vi "Orig_Channel Read Write.vi"() -> ()   [LabVIEW 2021, in "Template Test Helpers.lvlib"]
uses:
  <vilib>/CIF Foundation/CIF Core/CIFCore/Common/Typedef/gRPC Reported Plugin Status.ctl
  <vilib>/CIF Foundation/CIF Core/CIFCore/Common/Typedef/Plugin State.ctl
  <vilib>/CIF Foundation/CIF Core/CIFCore/Common/Typedef/Timing Statistics.ctl
  <vilib>/CIF Foundation/CIF Core/CIFCore/Common/Typedef/Timing Stats Base.ctl
  <vilib>/CIF Foundation/CIF Core/CIFCore/Common/Typedef/FIFO Statistics.ctl
  <vilib>/CIF Foundation/CIF Core/CIFCore/Common/Typedef/Simple Error.ctl
  <vilib>/CIF Foundation/CIF Core/CIFCore/Common/Typedef/Monitor Doubles.ctl
  <vilib>/CIF Foundation/CIF Core/CIFCore/Common/Typedef/Monitor U64.ctl
  <vilib>/CIF Foundation/CIF Core/CIFCore/Common/Typedef/Monitor I64.ctl
  <vilib>/CIF Foundation/CIF Channels Core/CIFChannels/Typedef/Direction.ctl
  <vilib>/CIF Foundation/CIF Core/CIFCore/Grpc/CIFCoreChannel_client/RPC Messages/cif_channelcore_ConnectSubscriber.ctl
  <vilib>/gRPC/LabVIEW gRPC Library/Client API/Close Client.vi
  <vilib>/CIF Foundation/CIF Channels Core/CIPC_Channels/Double/CIF_CIPC_Chn_Double.lvclass
  <vilib>/CIF Foundation/CIF Channels Core/CIPC_Channels/U64/CIF_CIPC_Chn_U64.lvclass
  Template Test Helpers.lvlib
  <vilib>/CIF Foundation/CIF Channels Core/CIFChannels/CIFChannels.lvclass
  <vilib>/CIF Foundation/CIF Core/CIFCore/Grpc/CIFCoreWrapper/CIFCoreWrapper.lvlib
  <vilib>/CIF Foundation/CIF Core/CIFCore/Grpc/CIFCoreChannel_client/CIFCoreChannel_client.lvlib
  <vilib>/CIF Foundation/CIF Core/CIFCore/Class/CIFCorePlugin.lvclass
  Common/Typedef/Channels.ctl
  Common/Template_Common.lvlib
  <vilib>/CIF Foundation/CIF Core/CIFCore/Class/Typedef/Energized States.ctl
  <vilib>/CIF Foundation/CIF Channels Core/ChannelCommon/typedef/New FIFO Instance Response.ctl
  <vilib>/CIF Foundation/CIF Channels Core/ChannelCommon/ChannelCommon.lvlib
  <vilib>/CIF Foundation/CIF Core/Channels/CIFChannelMng/CIFChannelMng.lvclass
  <vilib>/CIF Foundation/CIF Core/CIFCore/Common/CIFCoreCommon.lvlib
panel:
  out "Data 4":u64
  out "error out 4":errorcluster
  out "Node Status":T1 {"Monitor Doubles"."4" format="%#_9g"; "Monitor Doubles"."3" format="%#_9g"; "Monitor Doubles"."2" format="%#_9g"; "Monitor Doubles"."1" format="%#_9g"}
  in  "address":string="192.168.1.160:50051"
  in  "Data 3":dbl
  out "error out 3":errorcluster
  in  "stop":bool
  out "error out":errorcluster
  out "Data 2":dbl
  in  "Data":dbl
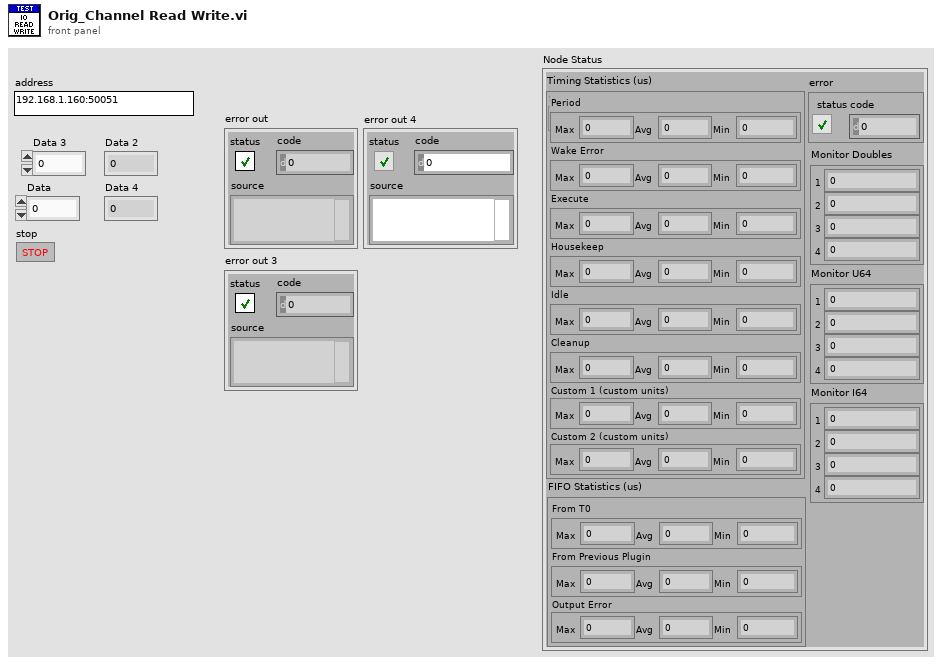
[diagram p1: front panel]
types:
  T1 = typedef "CIFCoreCommon.lvlib/gRPC Reported Plugin Status.ctl" = cluster{"State":T2, "Timing Statistics (us)":T3, "FIFO Statistics (us)":T5, "error":T6, "Monitor Doubles":T7, "Monitor U64":T8, "Monitor I64":T9}
  T2 = typedef "CIFCoreCommon.lvlib/Plugin State.ctl" = enum32{"Null", "Creating", "Listening", "Running", "CleaningUp", "Destroying"}
  T3 = typedef "CIFCoreCommon.lvlib/Timing Statistics.ctl" = cluster{"Period":T4, "Wake Error":T4, "Execute":T4, "Housekeep":T4, "Idle":T4, "Cleanup":T4, "Custom 1 (custom units)":T4, "Custom 2 (custom units)":T4}
  T4 = typedef "CIFCoreCommon.lvlib/Timing Stats Base.ctl" = cluster{"Max":i64, "Avg":dbl, "Min":i64}
  T5 = typedef "CIFCoreCommon.lvlib/FIFO Statistics.ctl" = cluster{"From T0":T4, "From Previous Plugin":T4, "Output Error":T4}
  T6 = typedef "CIFCoreCommon.lvlib/Simple Error.ctl" = cluster{"status":bool, "code":i32}
  T7 = typedef "CIFCoreCommon.lvlib/Monitor Doubles.ctl" = cluster{"1":dbl, "2":dbl, "3":dbl, "4":dbl}
  T8 = typedef "CIFCoreCommon.lvlib/Monitor U64.ctl" = cluster{"1":u64, "2":u64, "3":u64, "4":u64}
  T9 = typedef "CIFCoreCommon.lvlib/Monitor I64.ctl" = cluster{"1":i64, "2":i64, "3":i64, "4":i64}
  T10 = typedef "CIFCoreChannel_client.lvlib/cif_channelcore_ConnectSubscriber.ctl" = cluster{"subscriber_name":string, "publisher_name":string, "custom_connect":u8[]}
  T11 = typedef "CIFChannels.lvclass/Direction.ctl" = enum16{"Publisher", "Subscriber"}
  T12 = typedef "grpc-lvsupport-release.lvlib/grpcId.ctl" = u64
  T13 = typedef "Template_Common.lvlib/Channels.ctl" = enum16{"doubleout", "doublein1", "doublein2", "uint_out", "uint_in", "u8array_out", "u8array_in"}
  T14 = typedef "CIFCorePlugin.lvclass/Energized States.ctl" = enum16{"Listen", "Prepare", "Execute", "Housekeep", "Cleanup", "Destroy"}
  T15 = typedef "ChannelCommon.lvlib/New FIFO Instance Response.ctl" = cluster{"Publisher":string, "Custom Data":u8[]}
  T16 = typedef "Time_CIF_U.lvlib/Clock Conversion Map.ctl" = map{u8, cluster{"Last Reset":i64, "Offset Pair":T17, "Slope":dbl, "1/Slope":dbl}}
  T17 = typedef "Time_CIF_U.lvlib/Timestamp Pair.ctl" = cluster{"System Time":i64, "External Time":i64}
  T18 = typedef "CIFCoreCommon.lvlib/Channel Connection Data.ctl" = cluster{"Publisher Name":string, "Subscriber Name":string, "Connection Data":u8[]}
  T19 = typedef "CIFCoreCommon.lvlib/Channel Force Data.ctl" = cluster{"Channel Name":string, "Force Data":u8[], "Force Active":bool}
  T20 = typedef "CIFCoreCommon.lvlib/FIFO Publisher.ctl" = cluster{"Publisher Name":string, "New FIFO Instance Config":T21}
  T21 = typedef "ChannelCommon.lvlib/New FIFO Instance Configuration.ctl" = cluster{"Backpressure":bool, "Bytes/Message Override":u32, "Messages/FIFO Override":u32, "Custom Data":u8[]}
  T22 = typedef "CIFChannelMng.lvclass/FIFO Publisher Return.ctl" = cluster{"FIFO Instance Config":T15, "error":errorcluster, "Added":bool}
  T23 = typedef "CIFCoreChannel_client.lvlib/cif_channelcore_Channel.ctl" = cluster{"name":string, "direction":T24, "type":string, "custom_config":u8[], "connected":bool, "connected_name":string, "forced":bool, "channel_pattern":T25}
  T24 = typedef "CIFCoreChannel_client.lvlib/cif_channelcore_Direction.ctl" = enum32{"PUBLISHER", "SUBSCRIBER"}
  T25 = typedef "CIFCoreChannel_client.lvlib/cif_channelcore_PATTERN.ctl" = enum32{"UNKNOWN", "TAG", "FIFO", "MULTIFIFO", "BACKPRESSUREFIFO"}
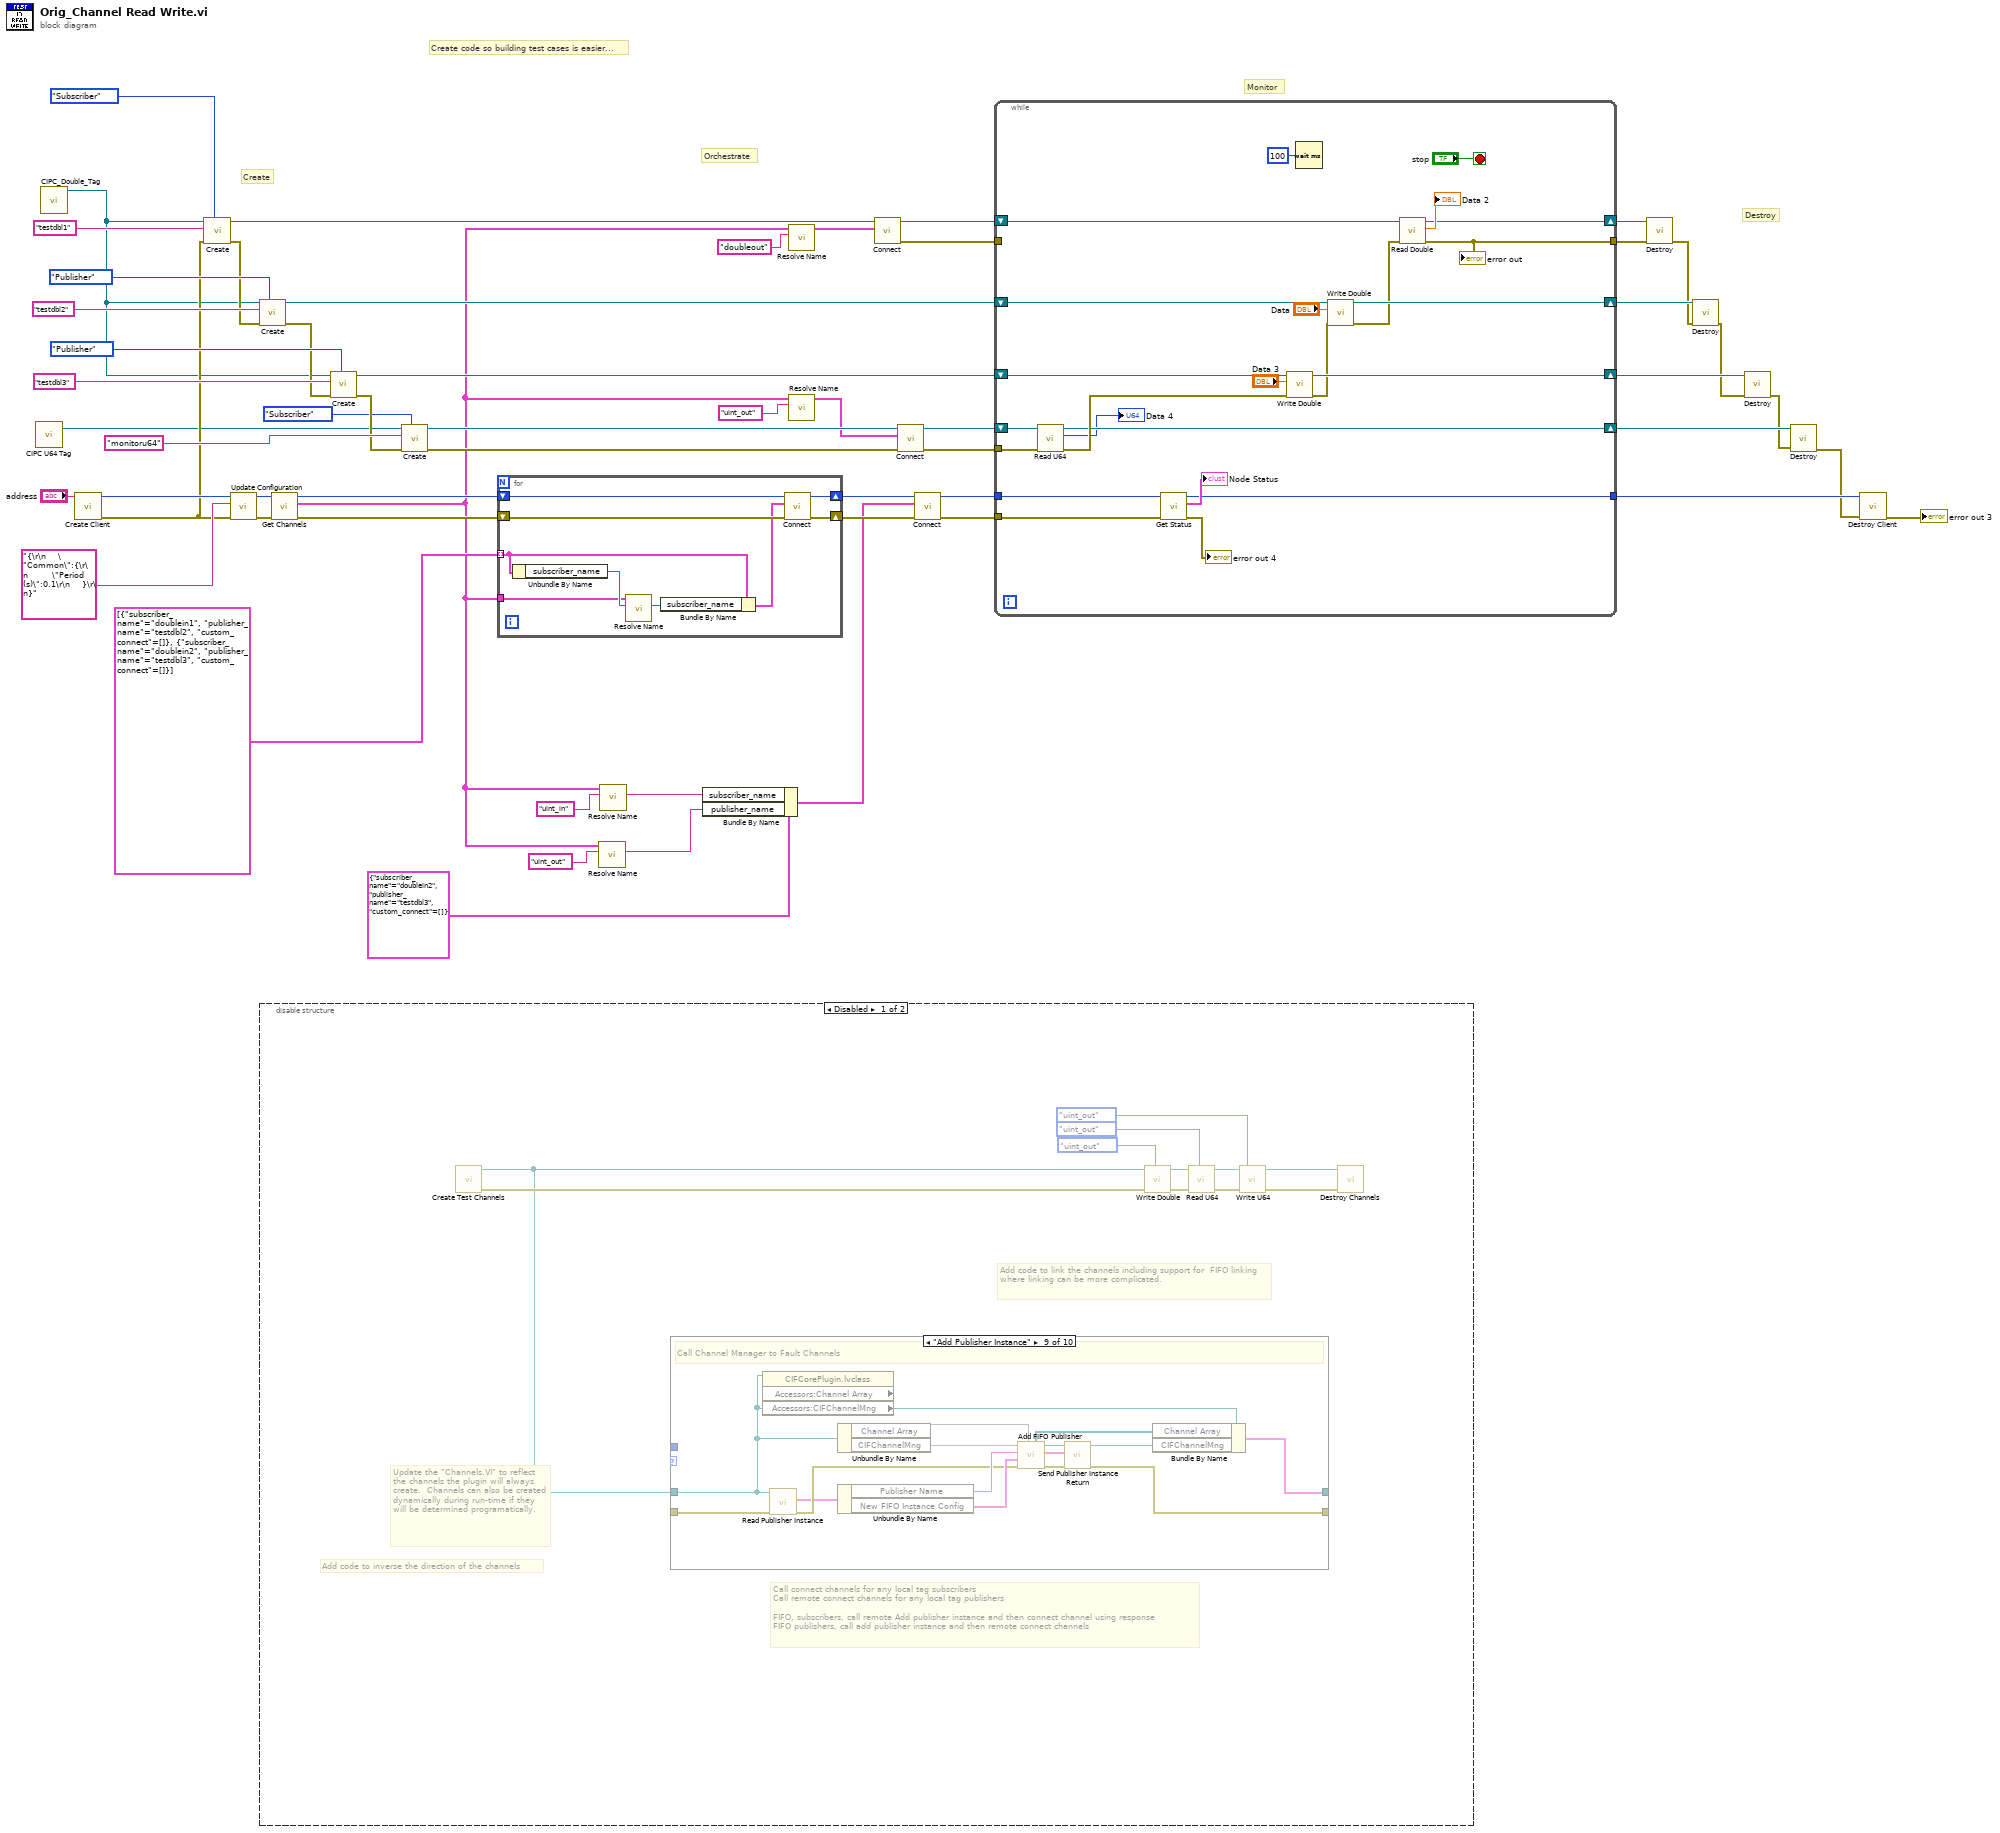
[diagram p0: block diagram]
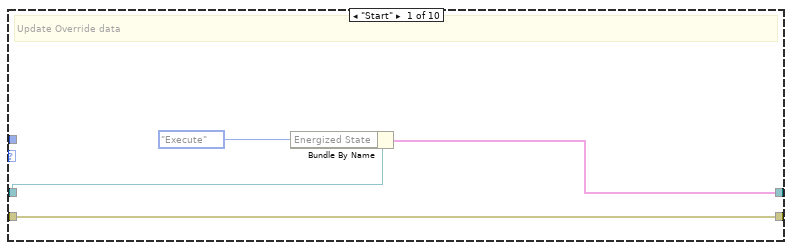
[diagram p2: hidden frame]
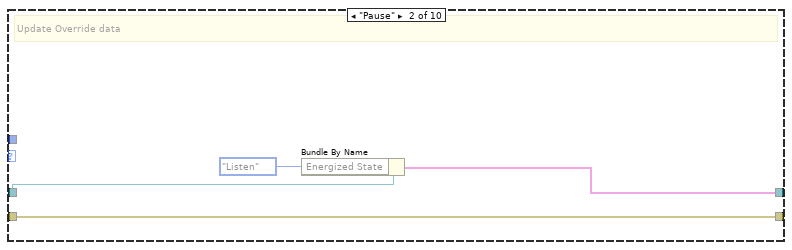
[diagram p3: hidden frame]
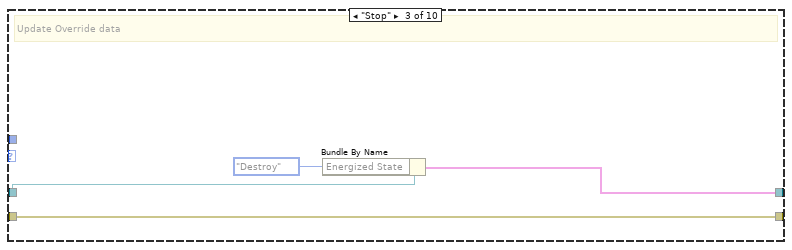
[diagram p4: hidden frame]
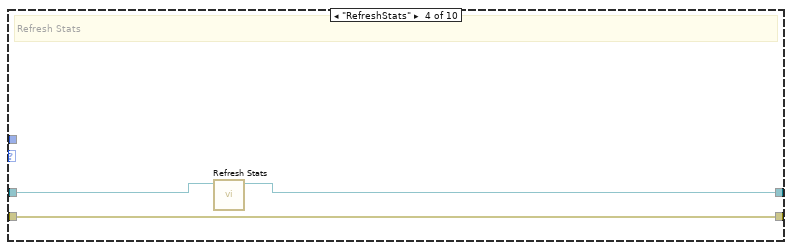
[diagram p5: hidden frame]
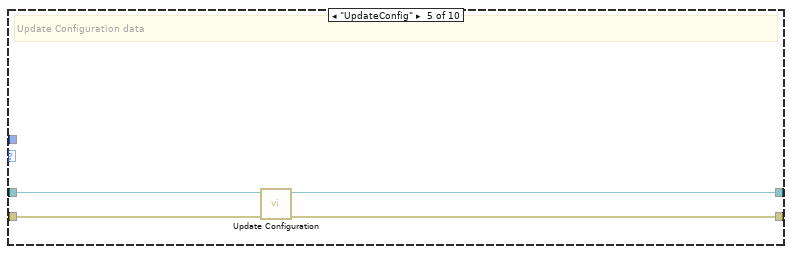
[diagram p6: hidden frame]
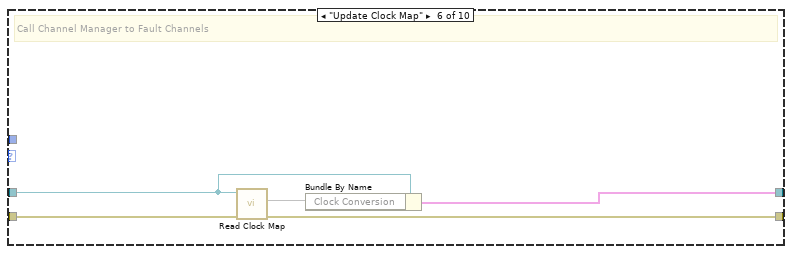
[diagram p7: hidden frame]
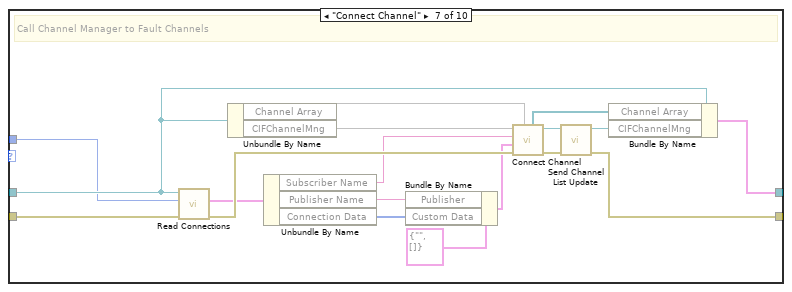
[diagram p8: hidden frame]
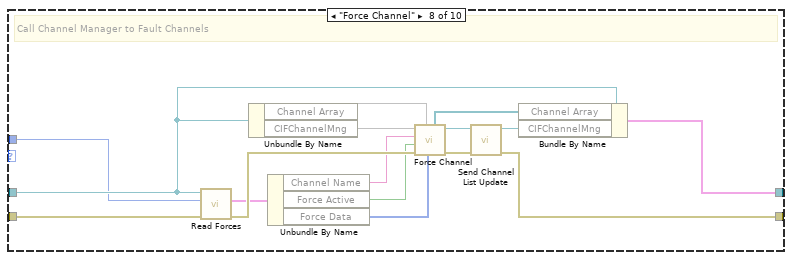
[diagram p9: hidden frame]
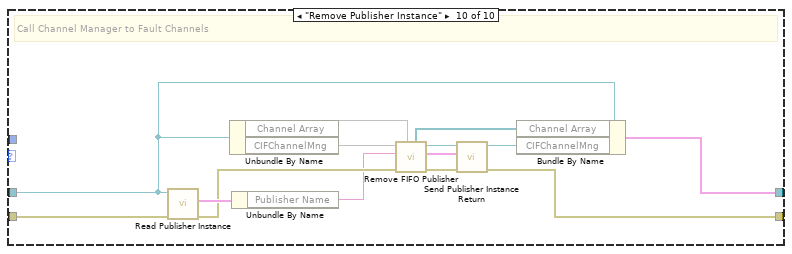
[diagram p10: hidden frame]
diagram:
  # "Create code so building test cases is easier..."
  # "Destroy"
  # "Monitor"
  # "Orchestrate"
  # "Create"
  n1 = call <vilib>:"CIPC U64 Tag.vi"() -> ("CIF_CIPC_Chn_U64.lvclass"=w2:refnum<class "CIF_CIPC_Chn_U64.lvclass">)  [unwired: 11 in]
  n2 = call <vilib>:"CIPC_Double_Tag.vi"() -> ("CIF_CIPC_Chn_Double.lvclass"=w1:refnum<class "CIF_CIPC_Chn_Double.lvclass">)  [unwired: 11 in]
  n3 = call <vilib>:"Create Client.vi"("address"="address") -> ("error out"=w24:errorcluster, "gRPC ID Out"=w25:T12)  [unwired: 9 in]
  n4 = call-dynamic "Create.vi"("Direction"=Direction."Subscriber", "error in (no error)"=w24, "Name"="testdbl1", "CIFTag in"=w1) -> ("error out"=w52:errorcluster, "CIFTag out"=w39:refnum<class "CIF_CIPC_Chn_Double.lvclass">)  [unwired: 6 in]
  n5 = call <vilib>:"Update Configuration.vi"("error in"=w24, "JSON Configuration"="{\r\n    \"Common\":{\r\n        \"Period (s)\":0.1\r\n    }\r\n}" ("JSON Configuration in"), "gRPC ID"=w25) -> ("error out"=w22:errorcluster, "gRPC ID out"=w23:T12)  [unwired: 7 in]
  n6 = call-dynamic "Create.vi"("Direction"=Direction."Publisher", "error in (no error)"=w52, "Name"="testdbl2", "CIFTag in"=w1) -> ("error out"=w43:errorcluster, "CIFTag out"=w55:refnum<class "CIF_CIPC_Chn_Double.lvclass">)  [unwired: 6 in]
  n7 = disable-structure shown="Disabled" {
    frame Disabled {
      # "Call connect channels for any local tag subscribers\nCall remote connect channels for any local tag publishers\n\nFIFO, subscribers, call remote Add publisher instance and then connect channel using response\nFIFO publishers, call add publisher instance and then remote connect channels"
      # "Add code to link the channels including support for  FIFO linking where linking can be more complicated."
      # "Add code to inverse the direction of the channels"
      # "Update the \"Channels.VI\" to reflect the channels the plugin will always create.  Channels can also be created dynamically during run-time if they will be determined programatically."
      n8 = call "Create Test Channels.vi"() -> ("error out"=w68:errorcluster, "CIFCorePlugin out"=w58:refnum<class "CIFCorePlugin.lvclass">)  [unwired: 10 in]
      n9 = case shown="\"Add Publisher Instance\"" {
        selector: _ -> [_ _ _ _ _ _ _ _ _ _]
        tunnel: _ -> [w69 w76 w80 w81 w86 w92 w109 w124 w138 w155]
        tunnel: w58 -> [w70 w75 w79 w83 w87 w88 w101 w113 w127 w142]
        tunnel: [w72 w74 w78 w82 w85 w91 w98 w112 w128 w143] -> _
        tunnel: [w69 w76 w80 w81 w84 w90 w104 w125 w129 w152] -> _
        tunnel: _ -> [_ _ _ _ _ _ w97 w111 _ _]
        frame "Start" {
          # "Update Override data"
          n10 = Bundle By Name(cluster=w70, "Energized State"=Energized_States."Execute" ("Energized States in")) -> (w72:cluster{})
        }
        frame "Pause" {
          # "Update Override data"
          n11 = Bundle By Name(cluster=w75, "Energized State"=Energized_States."Listen" ("Energized States in")) -> (w74:cluster{})
        }
        frame "Stop" {
          # "Update Override data"
          n12 = Bundle By Name(cluster=w79, "Energized State"=Energized_States."Destroy" ("Energized States in")) -> (w78:cluster{})
        }
        frame "RefreshStats" {
          # "Refresh Stats"
          n13 = call <vilib>:"Refresh Stats.vi"("CIFCorePlugin in"=w83) -> ("CIFCorePlugin out"=w82:refnum<class "CIFCorePlugin.lvclass">)  [unwired: 10 in]
        }
        frame "UpdateConfig" {
          # "Update Configuration data"
          n14 = call-dynamic <vilib>:"Update Configuration.vi"("error in (no error)"=w86, "CIFTemplateNode in"=w87) -> ("error out"=w84:errorcluster, "CIFTemplateNode out"=w85:refnum<class "CIFCorePlugin.lvclass">)  [unwired: 8 in]
        }
        frame "Update Clock Map" {
          # "Call Channel Manager to Fault Channels"
          n15 = call <vilib>:"Read Clock Map.vi"("error in"=w92, "CIFCorePlugin in"=w88) -> ("error out"=w90:errorcluster, "Clock Conversion"=w89:T16)  [unwired: 7 in, 1 out]
          n16 = Bundle By Name(cluster=w88, "Clock Conversion"=w89) -> (w91:cluster{})
        }
        frame "Connect Channel" {
          # "Call Channel Manager to Fault Channels"
          n17 = call <vilib>:"Read Connections.vi"("error in"=w109, "index"=w97, "CIFCorePlugin in"=w101) -> ("error out"=w105:errorcluster, "Connection"=w99:T18)  [unwired: 6 in, 1 out]
          n18 = Unbundle By Name(w101) -> ("Channel Array"=w103, "CIFChannelMng"=w110)
          n19 = Unbundle By Name(w99) -> ("Subscriber Name"=w100:string, "Publisher Name"=w95:string, "Connection Data"=w94:u8[])
          n20 = Bundle By Name(cluster=T15 {"Publisher"="", "Custom Data"=[]} ("Connection"), "Publisher"=w95, "Custom Data"=w94) -> (w93:T15)
          n21 = call <vilib>:"Connect Channel.vi"("Channel Array in"=w103, "error in (no error)"=w105, "Connection"=w93, "Subscriber Name"=w100, "CIFChannelMng in"=w110) -> ("error out"=w107:errorcluster, "CIFChannelMng out"=w108:refnum<class "CIFChannelMng.lvclass">, "Channel Array out"=w102:refnum<class "CIFChannels.lvclass">[])  [unwired: 3 in, 1 out]
          n22 = call <vilib>:"Send Channel List Update.vi"("error in (no error)"=w107, "CIFChannelMng in"=w108) -> ("error out"=w104:errorcluster, "CIFChannelMng out"=w106:refnum<class "CIFChannelMng.lvclass">)  [unwired: 8 in]
          n23 = Bundle By Name(cluster=w101, "Channel Array"=w102, "CIFChannelMng"=w106) -> (w98:cluster{})
        }
        frame "Force Channel" {
          # "Call Channel Manager to Fault Channels"
          n24 = call <vilib>:"Read Forces.vi"("error in"=w124, "index"=w111, "CIFCorePlugin in"=w113) -> ("error out"=w122:errorcluster, "Force"=w114:T19)  [unwired: 6 in, 1 out]
          n25 = Unbundle By Name(w113) -> ("Channel Array"=w119, "CIFChannelMng"=w123)
          n26 = Unbundle By Name(w114) -> ("Channel Name"=w117:string, "Force Active"=w116:bool, "Force Data"=w115:u8[])
          n27 = call <vilib>:"Force Channel.vi"("Force Data"=w115, "Channel Array in"=w119, "error in (no error)"=w122, "Force Active"=w116, "Channel Name"=w117, "CIFChannelMng in"=w123) -> ("error out"=w121:errorcluster, "CIFChannelMng out"=w120:refnum<class "CIFChannelMng.lvclass">, "Channel Array out"=w118:refnum<class "CIFChannels.lvclass">[])  [unwired: 2 in, 1 out]
          n28 = call <vilib>:"Send Channel List Update.vi"("error in (no error)"=w121, "CIFChannelMng in"=w120) -> ("error out"=w125:errorcluster, "CIFChannelMng out"=w126:refnum<class "CIFChannelMng.lvclass">)  [unwired: 8 in]
          n29 = Bundle By Name(cluster=w113, "Channel Array"=w118, "CIFChannelMng"=w126) -> (w112:cluster{})
        }
        frame "Add Publisher Instance" {
          # "Call Channel Manager to Fault Channels"
          n30 = property class="CIFCorePlugin.lvclass" props=["Accessors:Channel Array", "Accessors:CIFChannelMng"](reference=w127) -> ()  [unwired: 1 in, 4 out]
          n31 = call <vilib>:"Read Publisher Instance.vi"("error in"=w138, "CIFCorePlugin in"=w127) -> ("error out"=w137:errorcluster, "Publisher Instance"=w136:T20)  [unwired: 7 in, 1 out]
          n32 = Unbundle By Name(w127) -> ("Channel Array"=w132, "CIFChannelMng"=w141)
          n33 = Unbundle By Name(w136) -> ("Publisher Name"=w140:string, "New FIFO Instance Config"=w139:T21)
          n34 = call <vilib>:"Add FIFO Publisher.vi"("Channel Array in"=w132, "error in (no error)"=w137, "New FIFO Instance Config"=w139, "Channel Name"=w140, "CIFChannelMng in"=w141) -> ("error out"=w134:errorcluster, "FIFO Publisher"=w133:T22, "CIFChannelMng out"=w135:refnum<class "CIFChannelMng.lvclass">, "Channel Array out"=w131:refnum<class "CIFChannels.lvclass">[])  [unwired: 2 in, 1 out]
          n35 = call <vilib>:"Send Publisher Instance Return.vi"("error in (no error)"=w134, "Publisher Instance"=w133, "CIFChannelMng in"=w135) -> ("error out"=w129:errorcluster, "CIFChannelMng out"=w130:refnum<class "CIFChannelMng.lvclass">)  [unwired: 7 in]
          n36 = Bundle By Name(cluster=w127, "Channel Array"=w131, "CIFChannelMng"=w130) -> (w128:cluster{})
        }
        frame "Remove Publisher Instance" {
          # "Call Channel Manager to Fault Channels"
          n37 = call <vilib>:"Read Publisher Instance.vi"("error in"=w155, "CIFCorePlugin in"=w142) -> ("error out"=w150:errorcluster, "Publisher Instance"=w154:T20)  [unwired: 7 in, 1 out]
          n38 = Unbundle By Name(w142) -> ("Channel Array"=w145, "CIFChannelMng"=w151)
          n39 = Unbundle By Name(w154) -> ("Publisher Name"=w149:string)
          n40 = call <vilib>:"Remove FIFO Publisher.vi"("Channel Array in"=w145, "error in (no error)"=w150, "Channel Name"=w149, "CIFChannelMng in"=w151) -> ("error out"=w148:errorcluster, "FIFO Publisher"=w147:T22, "CIFChannelMng out"=w146:refnum<class "CIFChannelMng.lvclass">, "Channel Array out"=w144:refnum<class "CIFChannels.lvclass">[])  [unwired: 3 in, 1 out]
          n41 = call <vilib>:"Send Publisher Instance Return.vi"("error in (no error)"=w148, "Publisher Instance"=w147, "CIFChannelMng in"=w146) -> ("error out"=w152:errorcluster, "CIFChannelMng out"=w153:refnum<class "CIFChannelMng.lvclass">)  [unwired: 7 in]
          n42 = Bundle By Name(cluster=w142, "Channel Array"=w144, "CIFChannelMng"=w153) -> (w143:cluster{})
        }
      }
      n43 = call <vilib>:"Write Double.vi"("Channel Index"=Channels."uint_out" ("Channels"), "error in (no error)"=w68, "CIFCorePlugin in"=w58) -> ("error out"=w66:errorcluster, "CIFCorePlugin out"=w67:refnum<class "CIFCorePlugin.lvclass">)  [unwired: 7 in]
      n44 = call <vilib>:"Read U64.vi"("Channel Index"=Channels."uint_out" ("Channels"), "error in (no error)"=w66, "CIFCorePlugin in"=w67) -> ("error out"=w64:errorcluster, "CIFCorePlugin out"=w65:refnum<class "CIFCorePlugin.lvclass">)  [unwired: 6 in, 1 out]
      n45 = call <vilib>:"Write U64.vi"("Channel Index"=Channels."uint_out" ("Channels"), "error in (no error)"=w64, "CIFCorePlugin in"=w65) -> ("error out"=w62:errorcluster, "CIFCorePlugin out"=w63:refnum<class "CIFCorePlugin.lvclass">)  [unwired: 7 in]
      n46 = call <vilib>:"Destroy Channels.vi"("error in (no error)"=w62, "CIFCorePlugin in"=w63) -> ()  [unwired: 7 in, 3 out]
    }
    frame Enabled {
    }
  }
  n47 = call <vilib>:"Get Channels.vi"("error in"=w22, "gRPC ID"=w23) -> ("error out"=w21:errorcluster, "Channels"=w10:T23[], "gRPC ID out"=w20:T12)  [unwired: 7 in]
  n48 = call-dynamic "Create.vi"("Direction"=Direction."Publisher", "error in (no error)"=w43, "Name"="testdbl3", "CIFTag in"=w1) -> ("error out"=w34:errorcluster, "CIFTag out"=w45:refnum<class "CIF_CIPC_Chn_Double.lvclass">)  [unwired: 6 in]
  n49 = call-dynamic "Create.vi"("Direction"=Direction."Subscriber", "error in (no error)"=w34, "Name"="monitoru64", "CIFTag in"=w2) -> ("error out"=w31:errorcluster, "CIFTag out"=w33:refnum<class "CIF_CIPC_Chn_U64.lvclass">)  [unwired: 6 in]
  n50 = for {
    tunnel: T10[] [{"subscriber_name"="doublein1", "publisher_name"="testdbl2", "custom_connect"=[]}, {"subscriber_name"="doublein2", "publisher_name"="testdbl3", "custom_connect"=[]}] -> [w159] mode=indexing
    shift-right: [w162] -> w15
    shift-left: w21 -> [w163]
    shift-right: [w161] -> w16
    shift-left: w20 -> [w164]
    tunnel: w10 -> [w158]
    n51 = Unbundle By Name(w159) -> ("subscriber_name"=w160:string)
    n52 = call <vilib>:"Resolve Name.vi"("Name in"=w160, "Channels"=w158) -> ("Name out"=w156:string)  [unwired: 8 in, 1 out]
    n53 = Bundle By Name(cluster=w159, "subscriber_name"=w156) -> (w157:T10)
    n54 = call <vilib>:"Connect.vi"("error in"=w163, "Connection"=w157, "gRPC ID"=w164) -> ("error out"=w162:errorcluster, "gRPC ID out"=w161:T12)  [unwired: 7 in]
  }
  n55 = call <vilib>:"Resolve Name.vi"("Name in"="uint_out" ("Name"), "Channels"=w10) -> ("Name out"=w4:string)  [unwired: 8 in, 1 out]
  n56 = call <vilib>:"Resolve Name.vi"("Name in"="uint_in" ("Name"), "Channels"=w10) -> ("Name out"=w3:string)  [unwired: 8 in, 1 out]
  n57 = Bundle By Name(cluster=T10 {"subscriber_name"="doublein2", "publisher_name"="testdbl3", "custom_connect"=[]} ("Connection"), "subscriber_name"=w3, "publisher_name"=w4) -> (w12:T10)
  n58 = call <vilib>:"Resolve Name.vi"("Name in"="doubleout" ("Connection Name"), "Channels"=w10) -> ("Connection"=w9:T15)  [unwired: 8 in, 1 out]
  n59 = call <vilib>:"Resolve Name.vi"("Name in"="uint_out" ("Connection Name"), "Channels"=w10) -> ("Connection"=w19:T15)  [unwired: 8 in, 1 out]
  n60 = call-dynamic <vilib>:"Connect.vi"("Connection"=w9, "CIFTag in"=w39) -> ("error out"=w11:errorcluster, "CIFTag out"=w38:refnum<class "CIF_CIPC_Chn_Double.lvclass">)  [unwired: 8 in]
  n61 = call-dynamic <vilib>:"Connect.vi"("error in (no error)"=w31, "Connection"=w19, "CIFTag in"=w33) -> ("error out"=w30:errorcluster, "CIFTag out"=w32:refnum<class "CIF_CIPC_Chn_U64.lvclass">)  [unwired: 7 in]
  n62 = call <vilib>:"Connect.vi"("error in"=w15, "Connection"=w12, "gRPC ID"=w16) -> ("error out"=w13:errorcluster, "gRPC ID out"=w14:T12)  [unwired: 7 in]
  n63 = while {
    shift-right: [w185] -> w51
    shift-left: w38 -> [w175]
    shift-right: [w184] -> w50
    shift-left: w55 -> [w188]
    tunnel: [w182] -> w49
    shift-right: [w179] -> w47
    shift-left: w45 -> [w177]
    tunnel: w14 -> [w173]
    tunnel: w13 -> [w172]
    tunnel: [w170] -> w37
    tunnel: w30 -> [w168]
    shift-right: [w166] -> w29
    shift-left: w32 -> [w169]
    tunnel: w11 -> [_]
    stop <- "stop" stop-if-true
    n64 = call-dynamic <vilib>:"Read U64.vi"("error in (no error)"=w168, "CIFTag in"=w169) -> ("error out"=w167:errorcluster, "Data"=→"Data 4":u64, "CIFTag out"=w166:refnum<class "CIF_CIPC_Chn_U64.lvclass">)  [unwired: 6 in, 1 out]
    n65 = call <vilib>:"Get Status.vi"("error in"=w172, "gRPC ID"=w173) -> ("error out"=→"error out 4":errorcluster, "Node Status"=→"Node Status":T1, "gRPC ID out"=w170:T12)  [unwired: 7 in]
    n66 = call-dynamic <vilib>:"Write Double.vi"("error in (no error)"=w167, "Data"="Data 3", "CIFTag in"=w177) -> ("error out"=w176:errorcluster, "CIFTag out"=w179:refnum<class "CIF_CIPC_Chn_Double.lvclass">)  [unwired: 6 in, 1 out]
    n67 = Wait (ms)(milliseconds to wait=u32 100) -> ()  [unwired: 1 out]
    n68 = call-dynamic <vilib>:"Write Double.vi"("error in (no error)"=w176, "Data"="Data", "CIFTag in"=w188) -> ("error out"=w183:errorcluster, "CIFTag out"=w184:refnum<class "CIF_CIPC_Chn_Double.lvclass">)  [unwired: 6 in, 1 out]
    n69 = call-dynamic "Read Double.vi"("error in (no error)"=w183, "CIFTag in"=w175) -> ("error out"=w182:errorcluster, "Data"=→"Data 2":dbl, "CIFTag out"=w185:refnum<class "CIF_CIPC_Chn_Double.lvclass">)  [unwired: 6 in, 1 out]
    "error out" <- w182
  }
  n70 = call-dynamic "Destroy.vi"("error in (no error)"=w49, "CIFTag in"=w51) -> ("error out"=w48:errorcluster)  [unwired: 8 in, 1 out]
  n71 = call-dynamic "Destroy.vi"("error in (no error)"=w48, "CIFTag in"=w50) -> ("error out"=w42:errorcluster)  [unwired: 8 in, 1 out]
  n72 = call-dynamic "Destroy.vi"("error in (no error)"=w42, "CIFTag in"=w47) -> ("error out"=w28:errorcluster)  [unwired: 8 in, 1 out]
  n73 = call-dynamic "Destroy.vi"("error in (no error)"=w28, "CIFTag in"=w29) -> ("error out"=w27:errorcluster)  [unwired: 8 in, 1 out]
  n74 = call <vilib>:"Destroy Client.vi"("error in"=w27, "gRPC ID"=w37) -> ("error out"=→"error out 3":errorcluster)  [unwired: 9 in]
